vi "FGV_MultiLoopExit.vi"(10 "error in (no error)":errorcluster, 11 "Input":bool) -> (2 "Output":bool)   [LabVIEW 2017]
doc: "多循环并行退出。\n第一次调用，初始化移位寄存器为假。\n接收输入的状态量和错误簇。如果状态量为真或错误发生。保存真值至移位寄存器。并输出真值，停止当前循环。\n如果移位寄存器的值为真，输出真值，停止当前循环。"
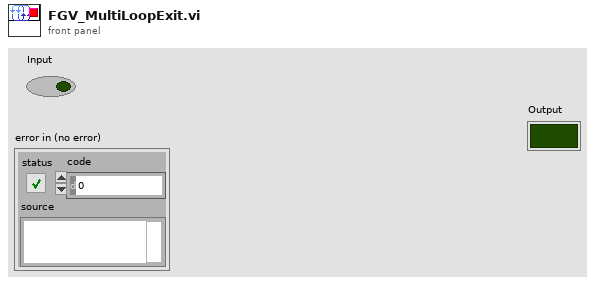
[diagram p1: front panel]
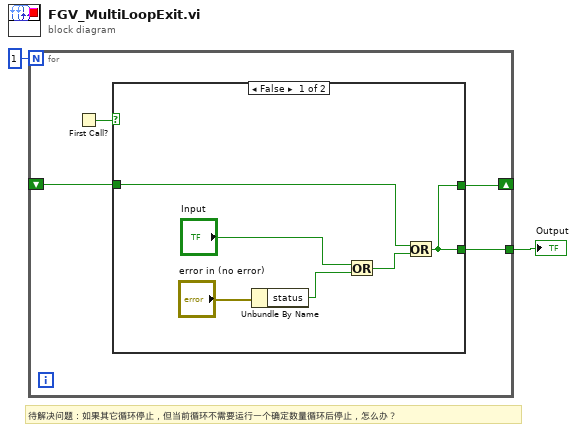
[diagram p0: block diagram]
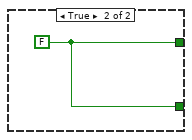
[diagram p2: hidden frame]
diagram:
  # "待解决问题：如果其它循环停止，但当前循环不需要运行一个确定数量循环后停止，怎么办？"
  n1 = for {
    N: 1 -> [_]
    shift-right: [w5] -> _
    shift-left: _ -> [w4]
    tunnel: [w3] -> w1
    n2 = First Call?() -> (First Call?: T/F=w6:bool)
    n3 = case shown="False" w6 {
      tunnel: [w7 w13] -> w5
      tunnel: w4 -> [w8 _]
      tunnel: [w7 w13] -> w3
      frame False {
        n4 = Unbundle By Name("error in (no error)") -> ("status"=w10:bool)
        n5 = Or(x="Input", y=w10) -> (x .or. y?=w9:bool)
        n6 = Or(x=w8, y=w9) -> (x .or. y?=w7:bool)
      }
      frame True {
        w13 = FALSE
      }
    }
  }
  "Output" <- w1
